vi "Describe Comparison.vi"(6 "Delta":variant, 8 "error in (no error)":errorcluster, 9 "Actual":variant, 10 "Expected":variant) -> (0 "error out":errorcluster, 2 "Description":string)   [LabVIEW 2020]
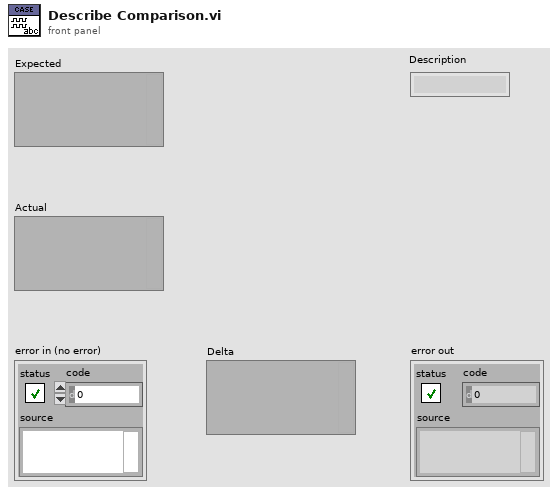
[diagram p1: front panel]
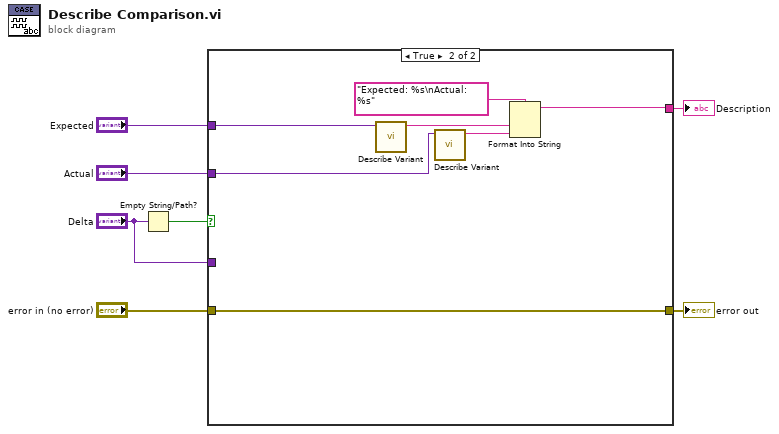
[diagram p0: block diagram]
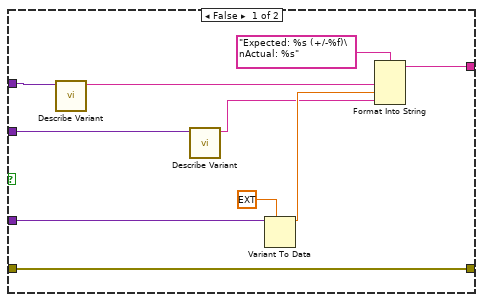
[diagram p2: hidden frame]
diagram:
  n1 = Empty String/Path?(string/path="Delta") -> (empty?=w3:bool)
  n2 = case shown="True" w3 {
    tunnel: "Expected" -> [w14 w21]
    tunnel: "Actual" -> [w12 w20]
    tunnel: "error in (no error)" -> [w8 w18]
    tunnel: [w8 w18] -> w4
    tunnel: "Delta" -> [w13 _]
    tunnel: [w11 w19] -> w1
    frame False {
      n3 = call "Describe Variant.vi"("Variant"=w14) -> ("Variant Description"=w15:string)  [unwired: 8 in, 2 out]
      n4 = call "Describe Variant.vi"("Variant"=w12) -> ("Variant Description"=w9:string)  [unwired: 8 in, 2 out]
      n5 = Variant To Data(type=ext 0.0, Variant=w13) -> (data=w10:ext)  [unwired: 1 in, 1 out]
      n6 = Format Into String(format string="Expected: %s (+/-%f)\nActual: %s", w15, w10, w9) -> (resulting string=w11:string)  [unwired: 2 in, 1 out]
    }
    frame True {
      n7 = call "Describe Variant.vi"("Variant"=w21) -> ("Variant Description"=w24:string)  [unwired: 8 in, 2 out]
      n8 = call "Describe Variant.vi"("Variant"=w20) -> ("Variant Description"=w22:string)  [unwired: 8 in, 2 out]
      n9 = Format Into String(format string="Expected: %s\nActual:   %s", w24, w22) -> (resulting string=w19:string)  [unwired: 2 in, 1 out]
    }
  }
  "Description" <- w1
  "error out" <- w4
